vi "OFDM_BitDetect.vi"(0 "Input symbols":cdb[](array[numeric]) format="%.2f", 1 "Modulation type":enum16{"QPSK(4QAM)", "64QAM", "16QAM", "BPSK"}(ring), 3 "error in (no error)":errorcluster) -> (7 "Output bits":i8[](array[numeric]), 10 "error out":errorcluster)   [LabVIEW 2018]
uses:
  <vilib>/addons/Modulation/Digital/General/MT Map QAM Symbols to Bits.vi
  <vilib>/addons/Modulation/Digital/General/MT Map PSK Symbols to Bits.vi
  <vilib>/addons/Modulation/niDMT.lvlib
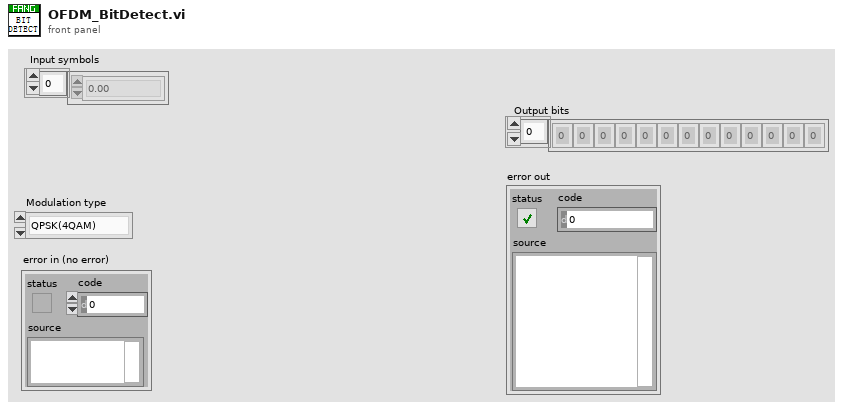
[diagram p1: front panel]
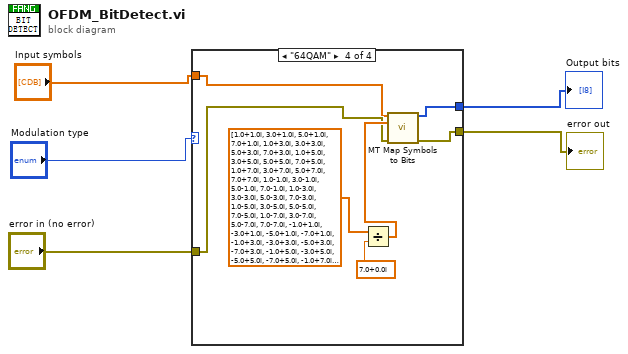
[diagram p0: block diagram]
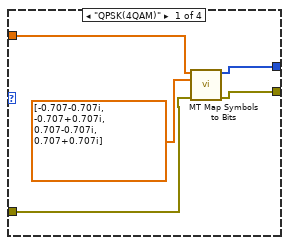
[diagram p2: hidden frame]
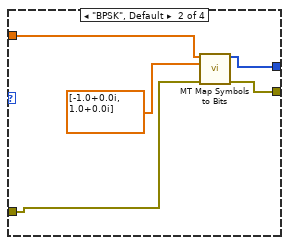
[diagram p3: hidden frame]
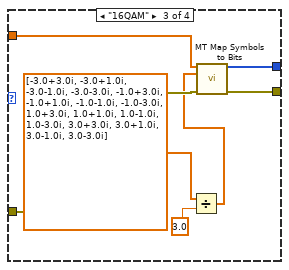
[diagram p4: hidden frame]
diagram:
  n1 = case shown="\"64QAM\"" "Modulation type" {
    tunnel: "Input symbols" -> [w10 w15 w22 w25]
    tunnel: "error in (no error)" -> [w8 w13 w21 w26]
    tunnel: [w6 w11 w20 w24] -> w2
    tunnel: [w7 w12 w19 w23] -> w1
    frame "QPSK(4QAM)" {
      n2 = call-poly <vilib>:"MT Map Symbols to Bits.vi"("symbols"=w10, "symbol map"=cdb[] [-0.707-0.707i, -0.707+0.707i, 0.707-0.707i, 0.707+0.707i], "error in (no error)"=w8) -> ("output bit stream"=w6:i8[], "error out"=w7:errorcluster)  [unwired: 11 in]
    }
    frame "BPSK", Default {
      n3 = call-poly <vilib>:"MT Map Symbols to Bits.vi"("symbols"=w15, "symbol map"=cdb[] [-1.0+0.0i, 1.0+0.0i], "error in (no error)"=w13) -> ("output bit stream"=w11:i8[], "error out"=w12:errorcluster)  [unwired: 11 in]
    }
    frame "16QAM" {
      n4 = Divide(x=cdb[] [-3.0+3.0i, -3.0+1.0i, -3.0-1.0i, -3.0-3.0i, -1.0+3.0i, -1.0+1.0i, -1.0-1.0i, -1.0-3.0i, 1.0+3.0i, 1.0+1.0i, 1.0-1.0i, 1.0-3.0i, 3.0+3.0i, 3.0+1.0i, 3.0-1.0i, 3.0-3.0i] ("symbol map"), y=3.0) -> (x/y=w16:cdb[])
      n5 = call-poly <vilib>:"MT Map Symbols to Bits.vi"("symbols"=w22, "symbol map"=w16, "error in (no error)"=w21) -> ("output bit stream"=w20:i8[], "error out"=w19:errorcluster)  [unwired: 11 in]
    }
    frame "64QAM" {
      n6 = Divide(x=cdb[] [1.0+1.0i, 3.0+1.0i, 5.0+1.0i, 7.0+1.0i, 1.0+3.0i, 3.0+3.0i, 5.0+3.0i, 7.0+3.0i, 1.0+5.0i, 3.0+5.0i, 5.0+5.0i, 7.0+5.0i, 1.0+7.0i, 3.0+7.0i, 5.0+7.0i, 7.0+7.0i, 1.0-1.0i, 3.0-1.0i, 5.0-1.0i, 7.0-1.0i, 1.0-3.0i, 3.0-3.0i, 5.0-3.0i, 7.0-3.0i, 1.0-5.0i, 3.0-5.0i, 5.0-5.0i, 7.0-5.0i, 1.0-7.0i, 3.0-7.0i, 5.0-7.0i, 7.0-7.0i, -1.0+1.0i, -3.0+1.0i, -5.0+1.0i, -7.0+1.0i, -1.0+3.0i, -3.0+3.0i, -5.0+3.0i, -7.0+3.0i, -1.0+5.0i, -3.0+5.0i, -5.0+5.0i, -7.0+5.0i, -1.0+7.0i, -3.0+7.0i, -5.0+7.0i, -7.0+7.0i, -1.0-1.0i, -3.0-1.0i, -5.0-1.0i, -7.0-1.0i, -1.0-3.0i, -3.0-3.0i, -5.0-3.0i, -7.0-3.0i, -1.0-5.0i, -3.0-5.0i, -5.0-5.0i, -7.0-5.0i, -1.0-7.0i, -3.0-7.0i, -5.0-7.0i, -7.0-7.0i] ("appended array"), y=cdb 7.0+0.0i) -> (x/y=w27:cdb[])
      n7 = call-poly <vilib>:"MT Map Symbols to Bits.vi"("symbols"=w25, "symbol map"=w27, "error in (no error)"=w26) -> ("output bit stream"=w24:i8[], "error out"=w23:errorcluster)  [unwired: 11 in]
    }
  }
  "Output bits" <- w2
  "error out" <- w1
